vi "Configure Data Log Measurement Range.vi"(6 "Data Log Auto Range (False)":bool, 7 "Data Log Measurement Range (0.0)":dbl format="%^.3e", 8 "error in (no error)":errorcluster {"code" format="%.0x"}, 9 "Data Log Type (1: Voltage)":i32(ring)=1 items=["Voltage"=1, "Current"=0], 10 "Channel Name (1)":string="1", 11 "VISA resource name":refnum<visa-resource-name>) -> (0 "error out":errorcluster {"code" format="%.0x"}, 3 "VISA resource name out":refnum<visa-resource-name>)   [LabVIEW 2010, in "Agilent N6700 Series.lvlib"]
doc: "Configures the measurement range of the data logger.\n\n<b>Note:</b>\n\nThis VI only applies to the N6705B DC Power Analyzer."
uses:
  Agilent N6700 Series.lvlib
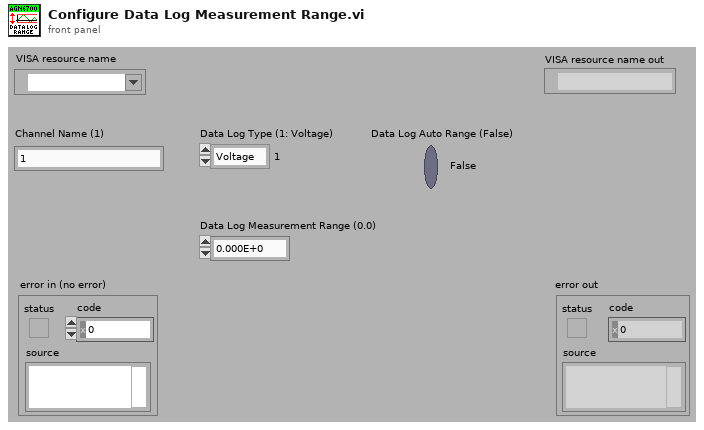
[diagram p1: front panel]
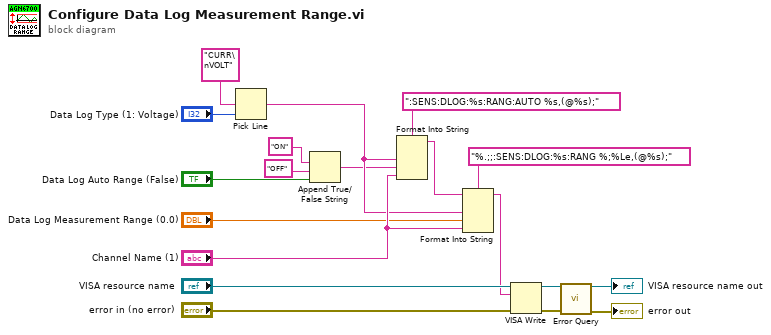
[diagram p0: block diagram]
diagram:
  n1 = Pick Line(multi-line string="CURR\nVOLT", line index="Data Log Type (1: Voltage)") -> (output string=w8:string)  [unwired: 1 in]
  n2 = Append True/False String(1:"Data Log Auto Range (False)", 2:"OFF", 3:"ON") -> (0:w3:string)  [unwired: 1 in]
  n3 = Format Into String(format string=":SENS:DLOG:%s:RANG:AUTO %s,(@%s);", w8, w3, "Channel Name (1)") -> (resulting string=w13:string)  [unwired: 2 in, 1 out]
  n4 = Format Into String(format string="%.;;:SENS:DLOG:%s:RANG %;%Le,(@%s);", initial string=w13, w8, "Data Log Measurement Range (0.0)", "Channel Name (1)") -> (resulting string=w12:string)  [unwired: 1 in, 1 out]
  n5 = VISA Write(VISA resource name="VISA resource name", write buffer=w12, error in (no error)="error in (no error)") -> (VISA resource name out=w15:refnum<visa-resource-name>, error out=w14:errorcluster)  [unwired: 1 out]
  n6 = call "Error Query.vi"("VISA resource name"=w15, "error in (no error)"=w14) -> ("VISA resource name out"=→"VISA resource name out":refnum<visa-resource-name>, "error out"=→"error out":errorcluster)  [unwired: 10 in, 2 out]
